vi "Keithley 2450 Read Single.vi"() -> ()   [LabVIEW 2015]
doc: "This example shows how to configure a measurement and take a reading."
uses:
  <instrlib>/Keithley 2450/Keithley 2450.lvlib
panel:
  in  "error in (no error)":errorcluster
  in  "Source Mode  (0: Voltage)":u16(ring) items=["Voltage", "Current"]
  in  "Compliance Level (0.1)":dbl=0.1
  in  "Output Level (0)":dbl
  out "Resistance (ohm)":dbl
  out "Current (A)":dbl
  out "Voltage (V)":dbl
  in  "VISA resource name":refnum<visa-resource-name>
  # "(c) 2006 National Instruments.  ALL RIGHTS RESERVED."
  # "Source Settings"
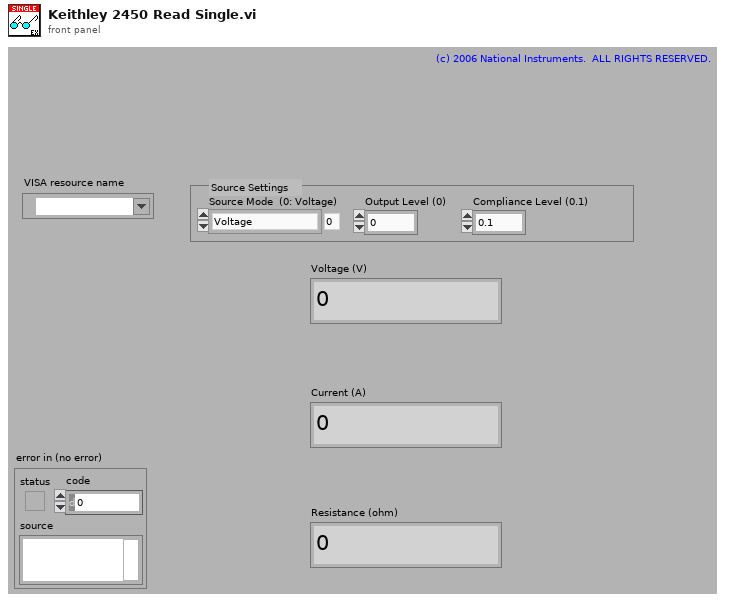
[diagram p1: front panel]
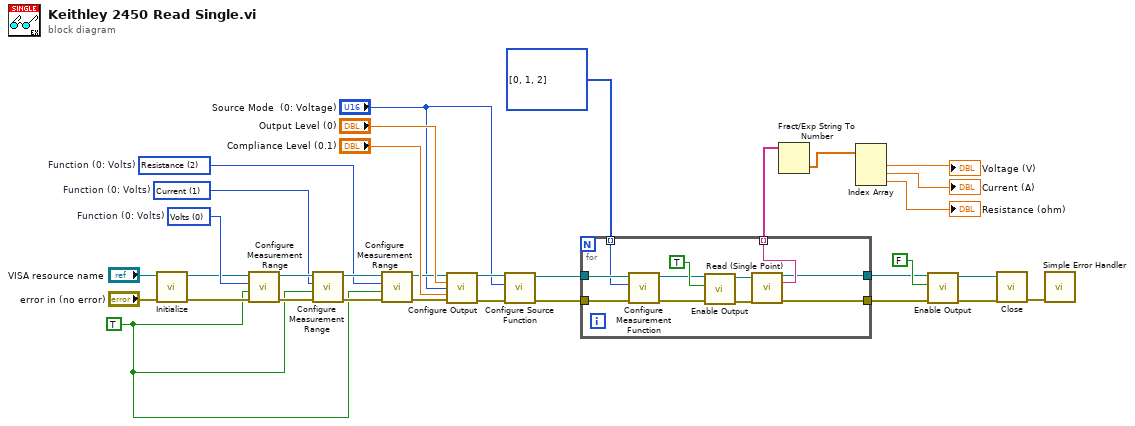
[diagram p0: block diagram]
diagram:
  w1 = TRUE ("Enable Output (T: Enable)")
  w7 = u16[] [0, 1, 2] items=["Volts", "Current", "Auto Resistance"]
  w25 = u16 2 items=["Volts", "Current", "Resistance"]  # Function (0: Volts)
  w26 = u16 1 items=["Volts", "Current", "Resistance"]  # Function (0: Volts)
  w27 = u16 0 items=["Volts", "Current", "Resistance"]  # Function (0: Volts)
  n1 = call <instrlib>:"Initialize.vi"("error in (no error)"="error in (no error)", "VISA resource name"="VISA resource name") -> ("error out"=w18:errorcluster, "VISA resource name out"=w19:refnum<visa-resource-name>)  [unwired: 8 in]
  n2 = call <instrlib>:"Configure Measurement Range.vi"("error in (no error)"=w18, "Enable Auto Range (T:Enable)"=w1, "Function (0: Volts)"=w27, "VISA resource name"=w19) -> ("error out"=w30:errorcluster, "VISA resource name out"=w31:refnum<visa-resource-name>)  [unwired: 6 in]
  n3 = call <instrlib>:"Configure Measurement Range.vi"("error in (no error)"=w30, "Enable Auto Range (T:Enable)"=w1, "Function (0: Volts)"=w26, "VISA resource name"=w31) -> ("error out"=w29:errorcluster, "VISA resource name out"=w28:refnum<visa-resource-name>)  [unwired: 6 in]
  n4 = call <instrlib>:"Configure Measurement Range.vi"("error in (no error)"=w29, "Enable Auto Range (T:Enable)"=w1, "Function (0: Volts)"=w25, "VISA resource name"=w28) -> ("error out"=w21:errorcluster, "VISA resource name out"=w20:refnum<visa-resource-name>)  [unwired: 6 in]
  n5 = call <instrlib>:"Configure Output.vi"("VISA resource name"=w20, "Source Level (0)"="Output Level (0)", "Source Mode  (0: Voltage)"="Source Mode  (0: Voltage)", "Source Limit Level (0.1)"="Compliance Level (0.1)", "error in (no error)"=w21) -> ("VISA resource name out"=w6:refnum<visa-resource-name>, "error out"=w5:errorcluster)  [unwired: 9 in]
  n6 = call <instrlib>:"Configure Source Function.vi"("error in (no error)"=w5, "Function (0: Volts)"="Source Mode  (0: Voltage)", "VISA resource name"=w6) -> ("error out"=w4:errorcluster, "VISA resource name out"=w3:refnum<visa-resource-name>)  [unwired: 7 in]
  n7 = for {
    tunnel: w3 -> [w44]
    tunnel: w4 -> [w43]
    tunnel: [w42] -> w12 mode=indexing
    tunnel: [w41] -> w14
    tunnel: [w40] -> w13
    tunnel: w7 -> [w39] mode=indexing
    n8 = call <instrlib>:"Configure Measurement Function.vi"("error in (no error)"=w43, "Function (0: Volts)"=w39, "VISA resource name"=w44) -> ("error out"=w36:errorcluster, "VISA resource name out"=w37:refnum<visa-resource-name>)  [unwired: 7 in]
    n9 = call <instrlib>:"Enable Output.vi"("error in (no error)"=w36, "Enable Output (T: Enable)"=TRUE, "VISA resource name"=w37) -> ("error out"=w35:errorcluster, "VISA resource name out"=w34:refnum<visa-resource-name>)  [unwired: 7 in]
    n10 = call <instrlib>:"Read (Single Point).vi"("VISA resource name"=w34, "error in (no error)"=w35) -> ("VISA resource name out"=w41:refnum<visa-resource-name>, "Data out"=w42:string, "error out"=w40:errorcluster)  [unwired: 11 in]
  }
  n11 = Fract/Exp String To Number(string=w12) -> (number=w11:dbl[])  [unwired: 3 in, 1 out]
  n12 = Index Array(array=w11) -> (element #1=→"Voltage (V)":dbl, element #2=→"Current (A)":dbl, element #3=→"Resistance (ohm)":dbl)  [unwired: 3 in]
  n13 = call <instrlib>:"Enable Output.vi"("error in (no error)"=w13, "Enable Output (T: Enable)"=FALSE, "VISA resource name"=w14) -> ("error out"=w15:errorcluster, "VISA resource name out"=w16:refnum<visa-resource-name>)  [unwired: 7 in]
  n14 = call <instrlib>:"Close.vi"("error in (no error)"=w15, "VISA resource name"=w16) -> ("error out"=w33:errorcluster)  [unwired: 9 in]
  n15 = call <vilib>:"Simple Error Handler.vi"("error in (no error)"=w33) -> ()  [unwired: 4 in, 5 out]
